vi "Diffrential (SubVI).vi"(11 "d(n)":dbl[](array[numeric])) -> (3 "d(n)-d(n+1)":dbl[](array[numeric]))   [LabVIEW 2017]
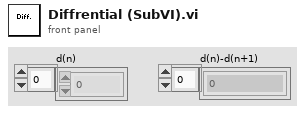
[diagram p1: front panel]
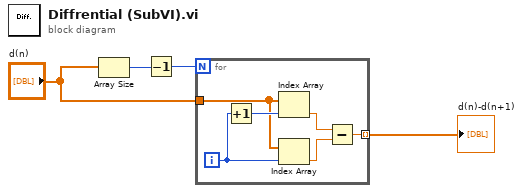
[diagram p0: block diagram]
diagram:
  n1 = Array Size(array="d(n)") -> (size(s)=w2:i32)
  n2 = Decrement(x=w2) -> (x-1=w1:i32)
  n3 = for {
    N: w1 -> [_]
    tunnel: [w8] -> w4 mode=indexing
    tunnel: "d(n)" -> [w7]
    i -> [w9]
    n4 = Increment(x=w9) -> (x+1=w10:i32)
    n5 = Index Array(array=w7, index=w10) -> (element=w6:dbl)
    n6 = Index Array(array=w7, index=w9) -> (element=w5:dbl)
    n7 = Subtract(x=w6, y=w5) -> (x-y=w8:dbl)
  }
  "d(n)-d(n+1)" <- w4
